vi "getNtpTime.vi"(0 "Time Server\nIP Address":string="10.100.2.20", 7 "error in (no error)":errorcluster) -> (20 "год":i32, 21 "месяц":i32, 22 "день месяца":i32, 23 "часы":i32, 24 "минуты":i32, 25 "секунды":i32, 26 "день недели":i32, 27 "error out":errorcluster)   [LabVIEW 2017]
doc: "Gets the time using the NTP protocol and sets the RT clock to that time"
panel:
  out "Time Server\nUsed":string
  out "Time Server\nRequested":string
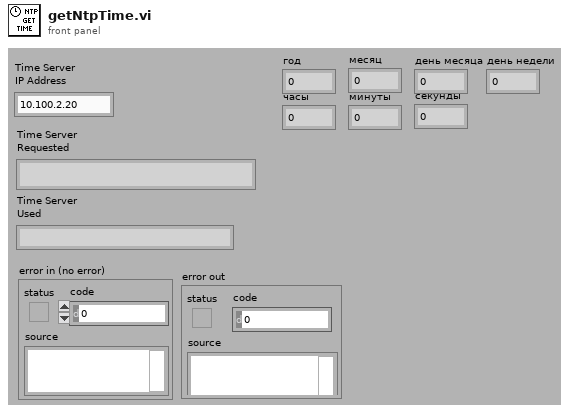
[diagram p1: front panel]
types:
  T1 = typedef "LVDateTimeRec.ctl" = cluster{"fractional second":dbl, "second":i32, "minute":i32, "hour":i32, "day of month":i32, "month":i32, "year":i32, "day of week":i32, "day of year":i32, "DST":i32}
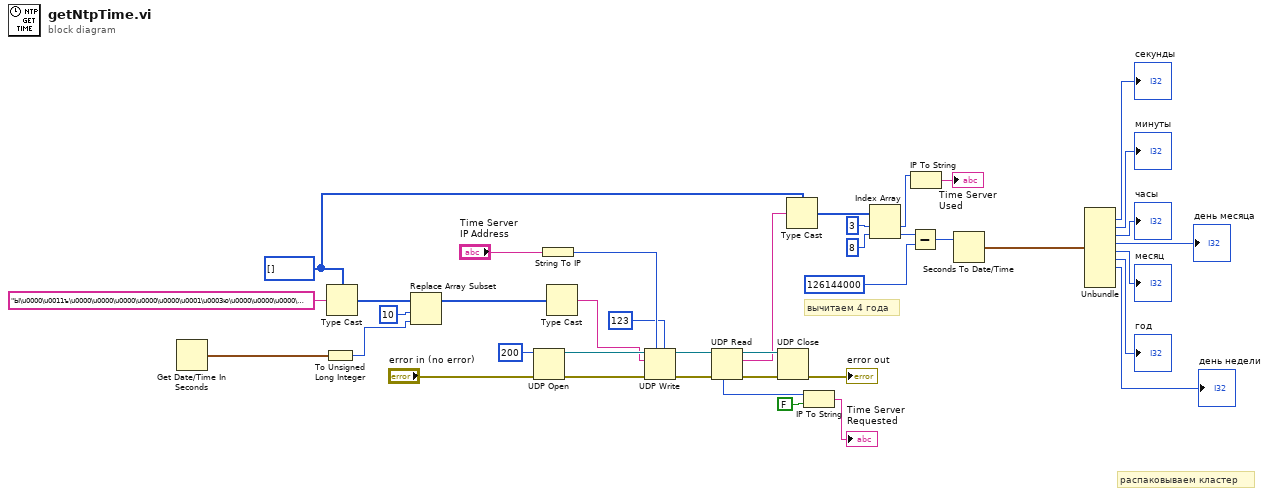
[diagram p0: block diagram]
diagram:
  w12 = u32[] []
  # "распаковываем кластер"
  # "вычитаем 4 года"
  n1 = Get Date/Time In Seconds() -> (seconds since 1Jan1904=w25:timestamp)
  n2 = To Unsigned Long Integer(number=w25) -> (unsigned 32bit integer=w11:u32)
  n3 = Type Cast(type=w12, x="Ы\u0000\u0011ъ\u0000\u0000\u0000\u0000\u0000\u0001\u0003ю\u0000\u0000\u0000\u0000Р!ъ*\u0017KЖ§\u0000\u0000\u0000\u0000\u0000\u0000\u0000\u0000\u0000\u0000\u0000\u0000\u0000\u0000\u0000\u0000Р'l\u001a‚MТсЂ:\u0000\u0000\u0000\u0000\u0000\u0000\u0000\u0000\u0000\u0000\u0000\u0000\u0000\u0000\u0000\u0000\u0000\u0000" ("String")) -> (*(type *) &x=w23:u32[])
  n4 = Replace Array Subset "Replace Array Subset"(array=w23, new element=w11, index=10) -> (w22:u32[])
  n5 = UDP Open(8:"error in (no error)", 11:u16 200 ("port")) -> (port=w38:refnum<k16>, 0:w39:errorcluster)  [unwired: 3 in, 1 out]
  n6 = String To IP(1:"Time Server\nIP Address") -> (0:w37:u32)
  n7 = Type Cast(x=w22) -> (*(type *) &x=w18:string)  [unwired: 1 in]
  n8 = UDP Write(address=w37, port or service name=u16 123 ("port"), connection ID=w38, data in=w18, 8:w39) -> (error out=w36:errorcluster, 3:w35:refnum<k16>)  [unwired: 1 in]
  n9 = UDP Read(connection ID=w35, 8:w36) -> (data out=w27:string, error out=w33:errorcluster, 3:w34:refnum<k16>, 6:w30:u32)  [unwired: 2 in, 1 out]
  n10 = UDP Close(connection ID=w34, 8:w33) -> (error out=→"error out":errorcluster)  [unwired: 1 out]
  n11 = Type Cast(type=w12, x=w27) -> (*(type *) &x=w26:u32[])
  n12 = IP To String(1:FALSE ("dot notation? (F)"), 2:w30) -> (0:→"Time Server\nRequested":string)
  n13 = Index Array(array=w26, index #1=3 ("index"), index #2=8 ("index")) -> (element #1=w16:u32, element #2=w10:u32)
  n14 = Subtract(x=w10, y=u32 126144000) -> (x-y=w17:u32)
  n15 = IP To String(2:w16) -> (0:→"Time Server\nUsed":string)  [unwired: 1 in]
  n16 = Seconds To Date/Time(time stamp (now)=w17) -> (date time rec=w8:T1)  [unwired: 1 in]
  n17 = Unbundle(w8) -> ("second"=→"секунды":i32, "minute"=→"минуты":i32, "hour"=→"часы":i32, "day of month"=→"день месяца":i32, "month"=→"месяц":i32, "year"=→"год":i32, "day of week"=→"день недели":i32)  [unwired: 3 out]
